vi "Teleop.vi"(10 "Match Info":T1={"Autonomous Elapsed Seconds"=0.0, "TeleOp Elapsed Seconds"=0.0, "Disabled Elapsed Seconds"=0.0, "Visited Autonomous"=FALSE, "Visited TeleOp"=FALSE, "Visited Disabled"=FALSE, "Autonomous Settings"={"Autonomous Style"=enum."Independent", "VI Refnum"=refnum}}, 11 "Call Context":T2) -> ()   [LabVIEW 2017]
doc: "This VI is called for each TeleOp packet received from the DS where the robot is not disabled. It is often used to read from the joysticks and update I/O or to update setpoints for timed control loops. It should complete and return within 20 milliseconds or it may miss DS packets."
uses:
  <vilib>/Rock Robotics/WPI/DriverStation/WPI_DriverStationDerivedRobotMode.ctl
  <vilib>/Rock Robotics/WPI/DriverStation/WPI_DriverStationMatch Info.ctl
  Public/Documents/Cross The Road Electronics/Phoenix-LabVIEW/Motor Controller/Controls/CTRE_Phoenix_MotorControl_FeedbackDevice.ctl
  Public/Documents/Cross The Road Electronics/Phoenix-LabVIEW/Motor Controller/Controls/CTRE_Phoenix_MotorControl_ControlMode.ctl
  Public/Documents/Cross The Road Electronics/Phoenix-LabVIEW/Motor Controller/Get/CTRE_Phoenix_MotorController_GetAnalogData.vi
  Public/Documents/Cross The Road Electronics/Phoenix-LabVIEW/Motor Controller/Get/CTRE_Phoenix_MotorController_GetClosedLoopData.vi
  Public/Documents/Cross The Road Electronics/Phoenix-LabVIEW/Motor Controller/Get/CTRE_Phoenix_MotorController_GetSelectedSensorData.vi
  Public/Documents/Cross The Road Electronics/Phoenix-LabVIEW/Motor Controller/Get/CTRE_Phoenix_MotorController_GetOutputCurrent_Enhanced.vi
  Public/Documents/Cross The Road Electronics/Phoenix-LabVIEW/Motor Controller/Get/CTRE_Phoenix_MotorController_GetVoltage.vi
panel:
  in  "Output":dbl
  in  "motionmagic?":bool
  out "Closed-loop Target":i32
  in  "Height 2":dbl
  out "Inches":dbl
  out "AnalogInVel":i32
  out "AnalogInWithOv":i32
  out "AnalogInRaw":i32
  out "Output Current":dbl
  in  "F":dbl=0.0095 format="%#_13g"
  in  "D":dbl format="%#_13g"
  in  "I":dbl format="%#_13g"
  in  "P":dbl format="%#_13g"
  out "Applied Throttle":dbl(graph)
  out "Closed-Loop Error":i32(graph)
  in  "Max Acceleration":i32=2000
  in  "Cruise Velocity":i32=2000
  out "Sensor Velocity":i32(graph)
  out "Sensor Position":cluster{"Height 2":dbl, dbl}(graph)
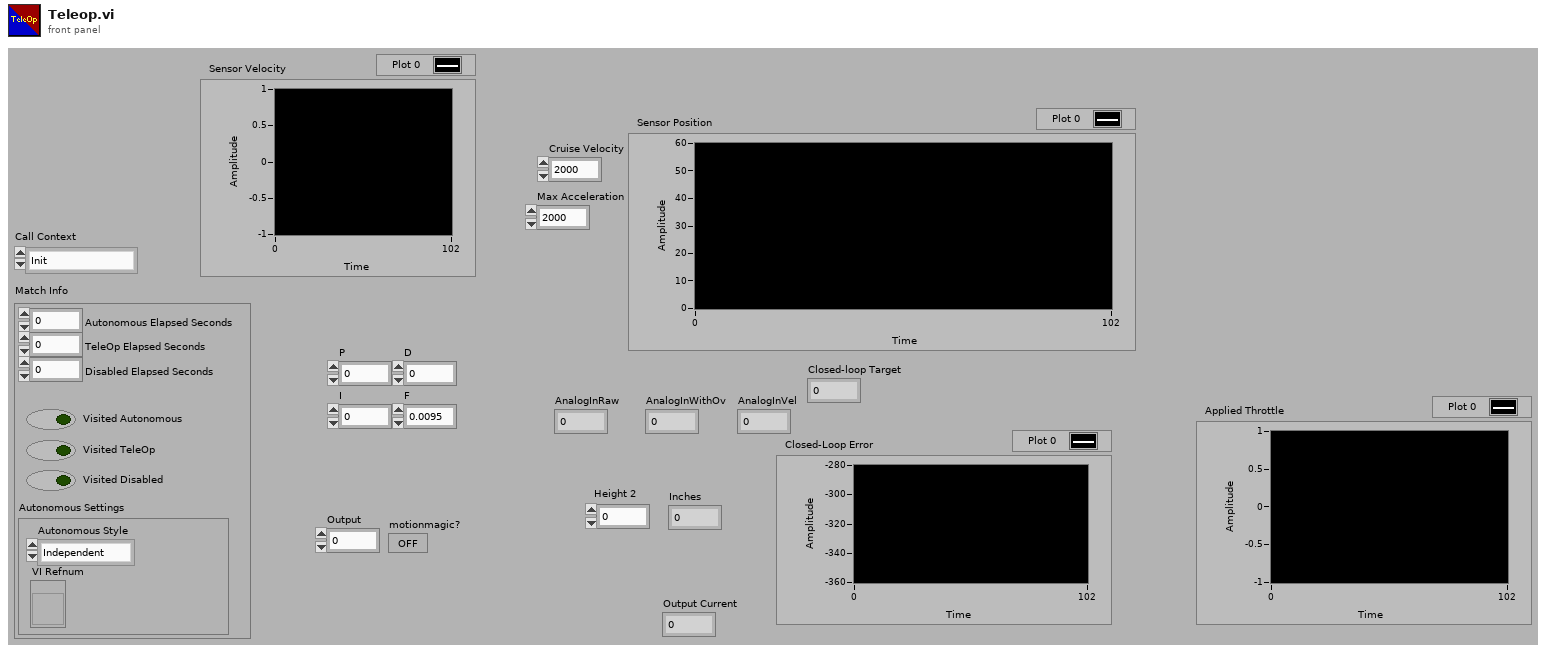
[diagram p1: front panel]
types:
  T1 = typedef "WPI_DriverStationMatch Info.ctl" = cluster{"Autonomous Elapsed Seconds":dbl, "TeleOp Elapsed Seconds":dbl, "Disabled Elapsed Seconds":dbl, "Visited Autonomous":bool, "Visited TeleOp":bool, "Visited Disabled":bool, "Autonomous Settings":cluster{"Autonomous Style":enum16{"Iterative", "Independent"}, "VI Refnum":refnum<vi>}}
  T2 = typedef "WPI_DriverStationDerivedRobotMode.ctl" = enum16{"Init", "Execute", "Stop"}
  T3 = typedef "CTRE_Phoenix_MotorControl_FeedbackDevice.ctl" = i8
  T4 = typedef "WPI_MotorControlDeviceRef.ctl" = cluster{"DeviceStatus":errorcluster, "Type":T5, "PWM":cluster{"PWM Channel":T6, "DeadBand":T7}, "CAN":cluster{"Device Number":u8, "SetOutput VI Ref":variant, "GetOutput VI Ref":variant, "Enable VI Ref":variant, "Disable VI Ref":variant, "Data":variant}, "Invert":bool, "DIO PWM":cluster{"PWM \"Enable\" Channel":T6, "DIOChannel":T8, "PWM Rate":dbl}}
  T5 = typedef "WPI_MotorControlType.ctl" = enum16{"PWM", "CAN", "DIO PWM"}
  T6 = typedef "FPGA_DIOPWMChannel.ctl" = enum8{"PWM 0", "PWM 1", "PWM 2", "PWM 3", "PWM 4", "PWM 5", "PWM 6", "PWM 7", "PWM 8", "PWM 9", "PWM MXP 0", "PWM MXP 1", "PWM MXP 2", "PWM MXP 3", "PWM MXP 4", "PWM MXP 5", "PWM MXP 6", "PWM MXP 7", "PWM MXP 8", "PWM MXP 9", "Invalid"}
  T7 = typedef "WPI_PWMDeadband.ctl" = cluster{"Name":string, "maxPositivePwm":i32, "minPositivePwm":i32, "centerPwm":i32, "maxNegativePwm":i32, "minNegativePwm":i32, "angularRange":u16}
  T8 = typedef "FPGA_DIOChannel.ctl" = enum8{"DIO 0", "DIO 1", "DIO 2", "DIO 3", "DIO 4", "DIO 5", "DIO 6", "DIO 7", "DIO 8", "DIO 9", "DIO MXP 0", "DIO MXP 1", "DIO MXP 2", "DIO MXP 3", "DIO MXP 4", "DIO MXP 5", "DIO MXP 6", "DIO MXP 7", "DIO MXP 8", "DIO MXP 9", "DIO MXP 10", "DIO MXP 11", "DIO MXP 12", "DIO MXP 13", "DIO MXP 14", "DIO MXP 15", "SPI Port CS1", "SPI Port CS2", "SPI Port CS3", "SPI Port MISO", "SPI Port MOSI", "Invalid"}
  T9 = typedef "CTRE_Phoenix_MotorControl_ControlMode.ctl" = u16
  T10 = typedef "WPI_JoystickDevRef.ctl" = cluster{"Device":T11}
  T11 = typedef "WPI_JoystickDeviceEnum.ctl" = enum16{"USB 0", "USB 1", "USB 2", "USB 3", "USB 4", "USB 5"}
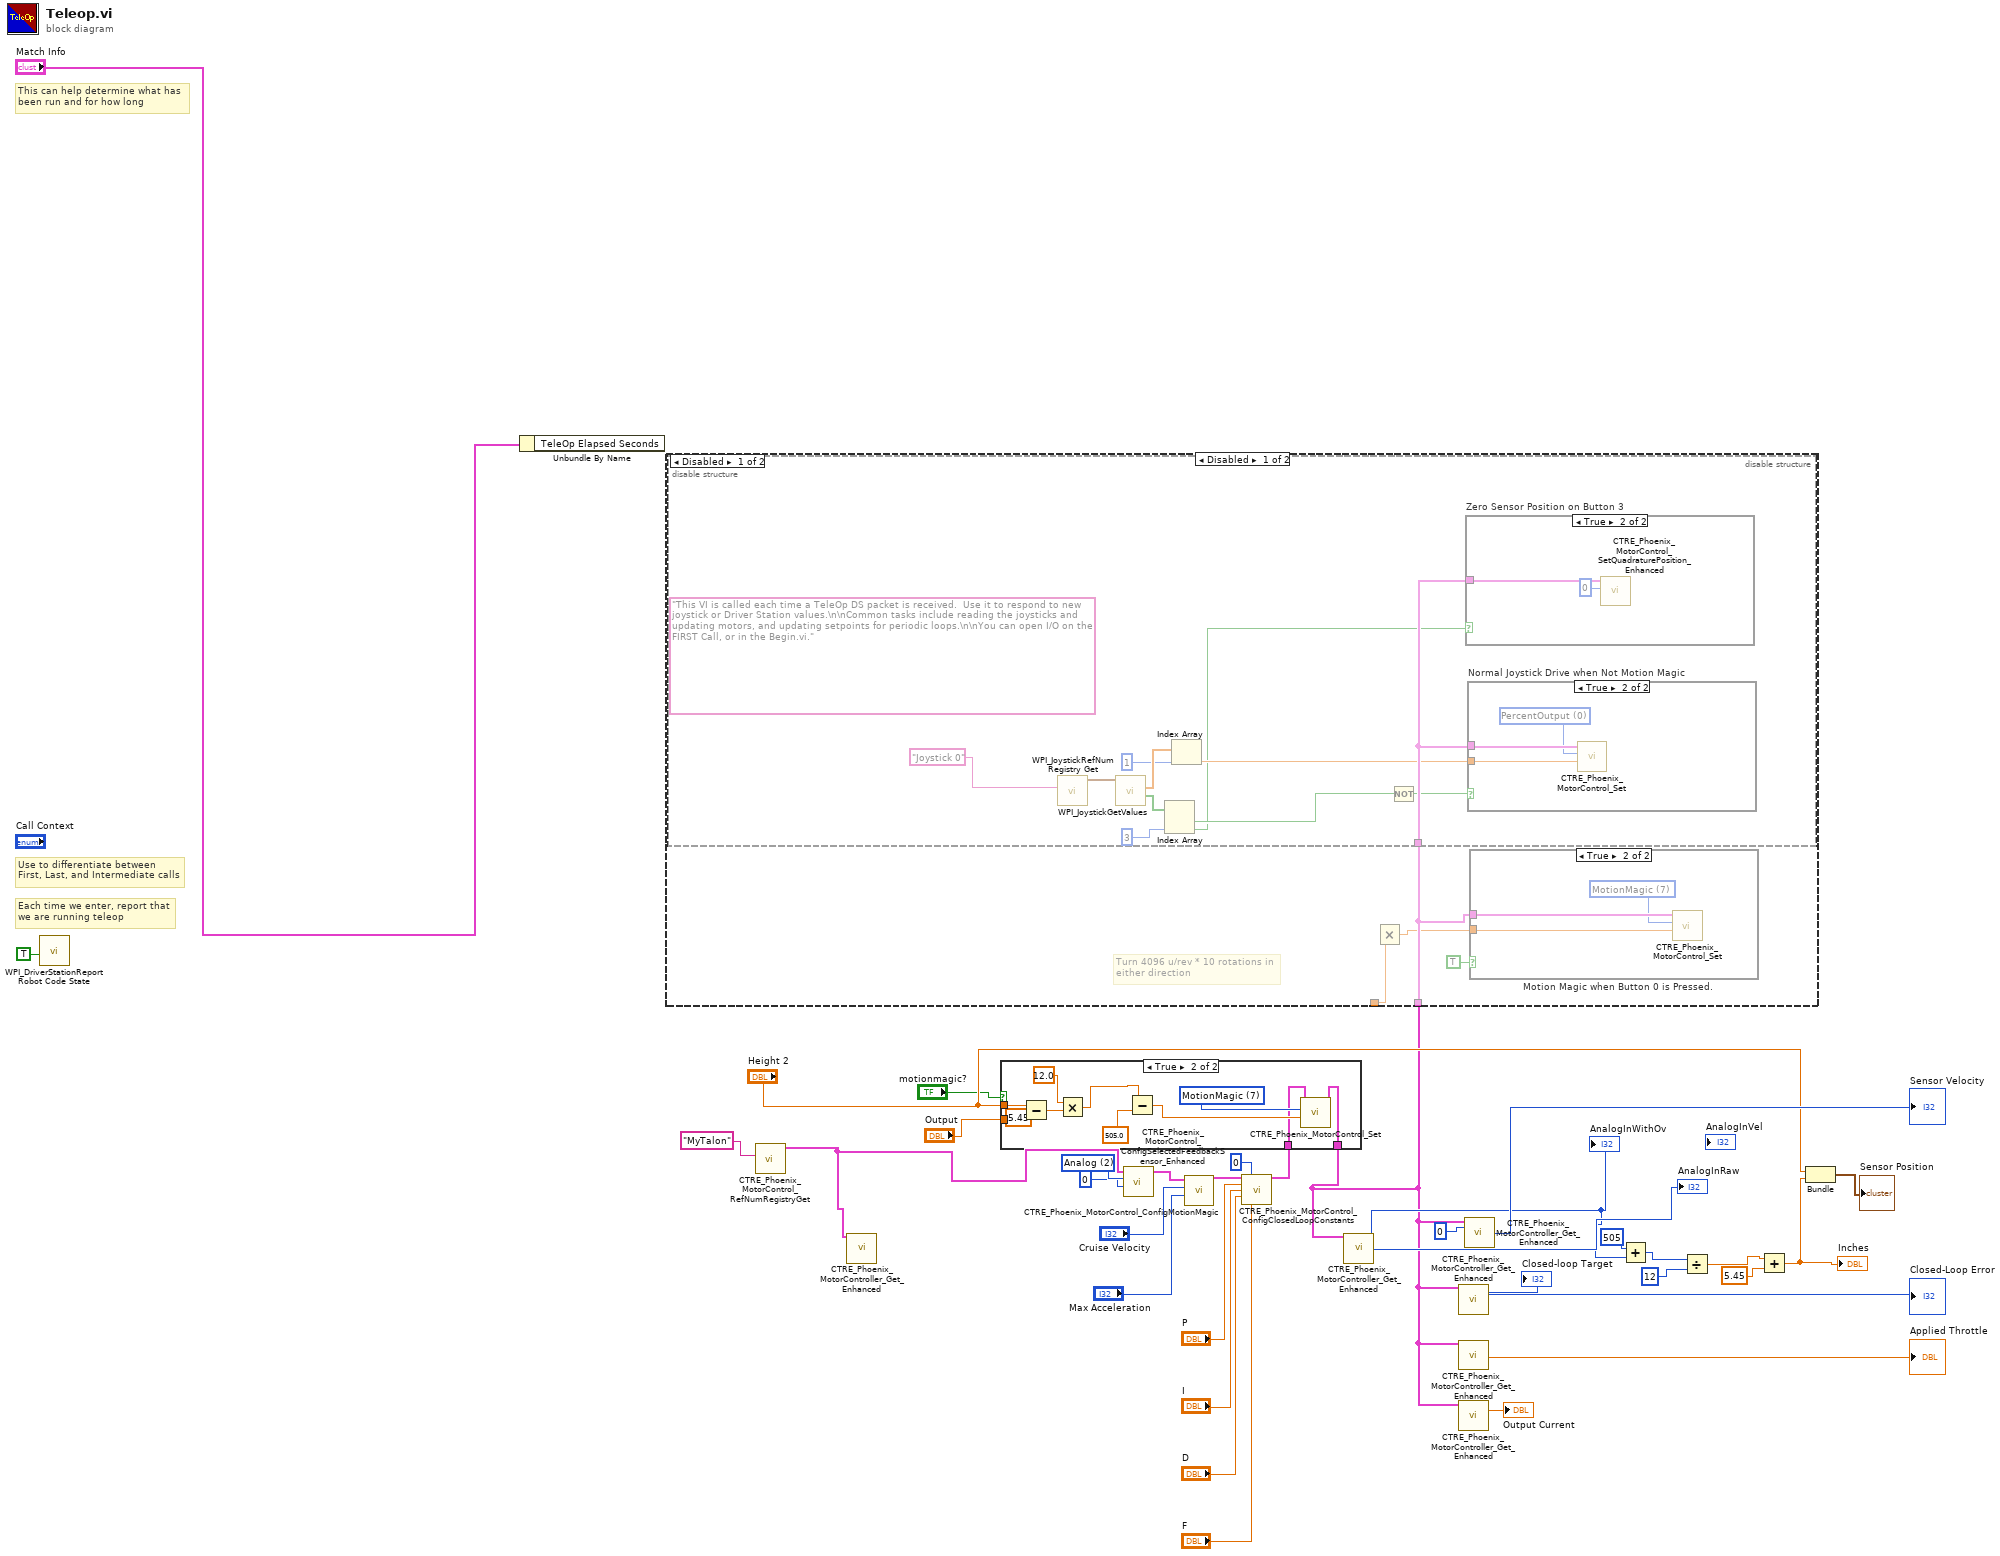
[diagram p0: block diagram]
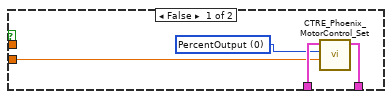
[diagram p2: hidden frame]
diagram:
  w32 = T3 2 items=["None"=-1, "QuadEncoder"=0, "Analog"=2, "Tachometer"=4, "Pulse Width Encoded Position"=8, "Sensor Sum (S0 + S1)"=9, "Sensor Difference (D0 - D1)"=10, "Remote Source 0"=11, "Remote Source 1"=12, "Software Emulated"=15] ("Feedback Device")
  # "Each time we enter, report that\nwe are running teleop"
  # "Use to differentiate between\nFirst, Last, and Intermediate calls"
  # "This can help determine what has\nbeen run and for how long"
  n1 = call <vilib>:"WPI_DriverStationReport Robot Code State.vi"("TeleOp"=TRUE ("Autonomous")) -> ()  [unwired: 10 in, 1 out]
  n2 = Unbundle By Name("Match Info") -> ()  [unwired: 1 out]
  n3 = call "CTRE_Phoenix_MotorControl_RefNumRegistryGet.vi"("refnum name"="MyTalon") -> ("PhoenixMotorControlDevRef"=w5:T4)  [unwired: 9 in, 1 out]
  n4 = call-poly "CTRE_Phoenix_MotorController_Get_Enhanced.vi"("PhoenixMotorControlDevRef"=w5) -> ()  [unwired: 10 in, 5 out]
  n5 = call "CTRE_Phoenix_MotorControl_ConfigSelectedFeedbackSensor_Enhanced.vi"("pidLoopIdx"=0, "Feedback Device"=w32, "PhoenixMotorControlDevRef"=w5) -> ("PhoenixMotorControlDevRef"=w31:T4)  [unwired: 7 in, 1 out]
  n6 = call "CTRE_Phoenix_MotorControl_ConfigMotionMagic.vi"("Acceleration"="Max Acceleration", "Cruise Velocity"="Cruise Velocity", "PhoenixMotorControlDevRef"=w31) -> ("PhoenixMotorControlDevRef"=w28:T4)  [unwired: 7 in, 1 out]
  n7 = call "CTRE_Phoenix_MotorControl_ConfigClosedLoopConstants.vi"("PhoenixMotorControlDevRef"=w28, "slotIdx"=0, "P"="P", "I"="I", "D"="D", "F"="F") -> ("PhoenixMotorControlDevRef"=w4:T4)  [unwired: 8 in, 1 out]
  n8 = case shown="True" "motionmagic?" {
    tunnel: "Height 2" -> [_ w44]
    tunnel: w4 -> [w38 w41]
    tunnel: [w39 w40] -> w3
    tunnel: "Output" -> [w36 _]
    frame False {
      w37 = T9 0 items=["PercentOutput"=0, "Position"=1, "Velocity"=2, "Current"=3, "Follower"=5, "MotionProfile"=6, "MotionMagic"=7, "MotionMagicArc"=8, "MotionProfileArc"=10, "Disabled"=15] ("Control Mode")
      n9 = call "CTRE_Phoenix_MotorControl_Set.vi"("Output"=w36, "Control Mode"=w37, "PhoenixMotorControlDevRef"=w38) -> ("PhoenixMotorControlDevRef"=w39:T4)  [unwired: 7 in, 1 out]
    }
    frame True {
      w49 = T9 7 items=["PercentOutput"=0, "Position"=1, "Velocity"=2, "Current"=3, "Follower"=5, "MotionProfile"=6, "MotionMagic"=7, "MotionMagicArc"=8, "MotionProfileArc"=10, "Disabled"=15] ("Control Mode")
      n10 = Subtract(x=w44, y=5.45) -> (x-y=w45:dbl)
      n11 = Multiply(x=12.0, y=w45) -> (x*y=w43:dbl)
      n12 = Subtract(x=w43, y=505.0) -> (x-y=w42:dbl)
      n13 = call "CTRE_Phoenix_MotorControl_Set.vi"("Output"=w42, "Control Mode"=w49, "PhoenixMotorControlDevRef"=w41) -> ("PhoenixMotorControlDevRef"=w40:T4)  [unwired: 7 in, 1 out]
    }
  }
  n14 = disable-structure shown="Disabled" {
    disable-tunnel: w3 -> [w54 _]
    disable-tunnel: _ -> [w50 _]
    frame Disabled {
      # "Turn 4096 u/rev * 10 rotations in\neither direction"
      n15 = disable-structure shown="Disabled" {
        disable-tunnel: w54 -> [w68 _]
        frame Disabled {
          (unwired) "This VI is called each time a TeleOp DS packet is received.  Use it to respond to new joystick or Driver Station values.\n\nCommon tasks include reading the joysticks and updating motors, and updating setpoints for periodic loops.\n\nYou can open I/O on the FIRST Call, or in the Begin.vi."
          n16 = call <vilib>:"WPI_JoystickRefNum Registry Get.vi"("refnum name"="Joystick 0") -> ("JoystickDevRef"=w66:T10)  [unwired: 1 in, 9 out]
          n17 = call <vilib>:"WPI_JoystickGetValues.vi"("JoystickDevRef"=w66) -> ("Buttons"=w65:bool[], "Axes"=w64:dbl[])  [unwired: 6 in, 3 out]
          n18 = Index Array(array=w65, index #2=3 ("index")) -> (element #1=w62:bool, element #2=w59:bool)  [unwired: 1 in]
          n19 = Index Array(array=w64, index=1) -> (element=w61:dbl)
          n20 = Not(x=w62) -> (.not. x?=w58:bool)
          n21 = case "Zero Sensor Position on Button 3" shown="True" w59 {
            tunnel: w68 -> [_ w70]
            frame False {
            }
            frame True {
              n22 = call "CTRE_Phoenix_MotorControl_SetQuadraturePosition_Enhanced.vi"("New Position"=0, "PhoenixMotorControlDevRef"=w70) -> ()  [unwired: 8 in, 2 out]
            }
          }
          n23 = case "Normal Joystick Drive when Not Motion Magic" shown="True" w58 {
            tunnel: w68 -> [_ w73]
            tunnel: w61 -> [_ w72]
            frame False {
            }
            frame True {
              w71 = T9 0 items=["PercentOutput"=0, "Position"=1, "Velocity"=2, "Follower"=5, "MotionProfile"=6, "MotionMagic"=7, "MotionMagicArc"=8, "TimedPercentOutput"=9, "Disabled"=15] ("Control Mode")
              n24 = call "CTRE_Phoenix_MotorControl_Set.vi"("Output"=w72, "Control Mode"=w71, "PhoenixMotorControlDevRef"=w73) -> ()  [unwired: 7 in, 2 out]
            }
          }
        }
        frame Enabled {
        }
      }
      n25 = Multiply(x=w50) -> (y=w52:dbl, x*y=w53:dbl)
      n26 = case "Motion Magic when Button 0 is Pressed." shown="True" TRUE {
        tunnel: w54 -> [_ w57]
        tunnel: w53 -> [_ w56]
        frame False {
        }
        frame True {
          w55 = T9 7 items=["PercentOutput"=0, "Position"=1, "Velocity"=2, "Follower"=5, "MotionProfile"=6, "MotionMagic"=7, "MotionMagicArc"=8, "TimedPercentOutput"=9, "Disabled"=15] ("Control Mode")
          n27 = call "CTRE_Phoenix_MotorControl_Set.vi"("Output"=w56, "Control Mode"=w55, "PhoenixMotorControlDevRef"=w57) -> ()  [unwired: 7 in, 2 out]
        }
      }
    }
    frame Enabled {
    }
  }
  n28 = call-poly "CTRE_Phoenix_MotorController_Get_Enhanced.vi"("PhoenixMotorControlDevRef"=w3) -> ("Position (Raw Sensor Units)"=w10:i32, "Velocity (Raw Sensor Units per 100 ms)"=→"AnalogInRaw":i32)  [unwired: 11 in, 2 out]
  "AnalogInWithOv" <- w10
  n29 = call-poly "CTRE_Phoenix_MotorController_Get_Enhanced.vi"("PhoenixMotorControlDevRef"=w3) -> ("Closed-loop Target"=→"Closed-loop Target":i32, "Closed-loop Error"=→"Closed-Loop Error":i32)  [unwired: 9 in, 4 out]
  n30 = call-poly "CTRE_Phoenix_MotorController_Get_Enhanced.vi"("PhoenixMotorControlDevRef"=w3) -> ("Percent Output"=→"Applied Throttle":dbl)  [unwired: 10 in, 4 out]
  n31 = call-poly "CTRE_Phoenix_MotorController_Get_Enhanced.vi"("PhoenixMotorControlDevRef"=w3) -> ("Output Current"=→"Output Current":dbl)  [unwired: 12 in, 2 out]
  n32 = call-poly "CTRE_Phoenix_MotorController_Get_Enhanced.vi"("PhoenixMotorControlDevRef"=w3, "pidLoopIdx"=u32 0) -> ("Velocity (Raw Sensor Units per 100 ms)"=→"Sensor Velocity":i32)  [unwired: 10 in, 3 out]
  n33 = Add(x=505, y=w10) -> (x+y=w16:i32)
  n34 = Divide(x=w16, y=12) -> (x/y=w13:dbl)
  n35 = Add(x=w13, y=5.45) -> (x+y=w9:dbl)
  "Inches" <- w9
  n36 = Bundle("Height 2"="Height 2", w9) -> (→"Sensor Position":cluster{"Height 2":dbl, dbl})  [unwired: 1 in]
